vi "Main.vi"(8 "error in":errorcluster, 9 "Error Queue":refnum<queue>, 11 "Application Events":refnum<user-event>) -> (0 "error out":errorcluster)   [LabVIEW 2020, in "Display Console.lvlib"]
doc: "VI Template with default error structure"
uses:
  Display Console.lvlib
  Error/Controls/Error Message Object.ctl
  Controller/Controls/Application Modules.ctl
  Error/Controls/Error Commands.ctl
  Controller/Controls/Application Event Object.ctl
  Controller/Controls/Application Events.ctl
  Controls/Operational Loop Commands.ctl
  Controls/Event Loop Data.ctl
  Controls/Operational Loop Data.ctl
  Controller/Controller.lvlib
  Error/Error Handler.lvlib
panel:
  out "Card Read":bool
  out "Message Screen":string
  out "Current Transaction":string
  # "[Covers: UI3B]"
  # "[Covers: UI3C]"
  # "[Covers: UI3]"
  # "[Covers: UI3A]"
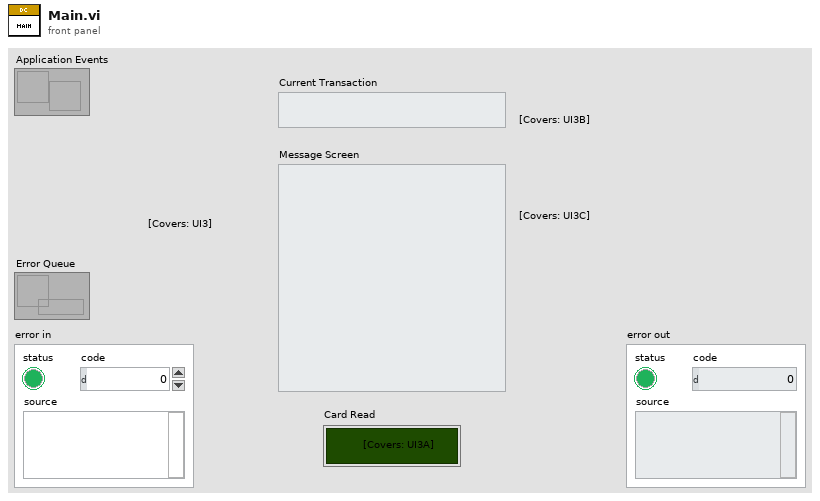
[diagram p1: front panel]
types:
  T1 = cluster{"Welcome Message":string, "Login Message":string, "Invalid Login Message":string, "Idle Message":string, "Terminate Session Message":string}
  T2 = typedef "Display Console.lvlib/Operational Loop Data.ctl" = cluster{"Current Module":T3}
  T3 = typedef "Controller.lvlib/Application Modules.ctl" = enum16{"Controller", "Error Module", "User Console", "Display Console", "Sensor Interface"}
  T4 = typedef "Display Console.lvlib/Event Loop Data.ctl" = cluster{"Current Module":T3, "Welcome Screen Messages":cluster{"Welcome Message":string, "Login Message":string, "Invalid Login Message":string, "Idle Message":string, "Terminate Session Message":string}}
  T5 = typedef "Controller.lvlib/Application Events.ctl" = enum16{"Terminate App", "Initialize", "New Transaction", "Balance Inquiry", "Balance Inquiry: Answer", "Deposit", "Deposit: Answer", "Withdrawal", "Withdrawal: Amount", "Fast Cash 50$", "Terminate Session", "Login", "Verify Account", "Invalid Login"}
  T6 = typedef "Display Console.lvlib/Operational Loop Commands.ctl" = enum16{"Shutdown"}
  T7 = enum16{"Load References", "Release References", "Get References"}
  T8 = typedef "Controller.lvlib/Controller Message Object.ctl" = cluster{"Commands":T9, "Source Module":T3, "Event Data":variant}
  T9 = typedef "Controller Commands.ctl" = enum16{"Shutdown"}
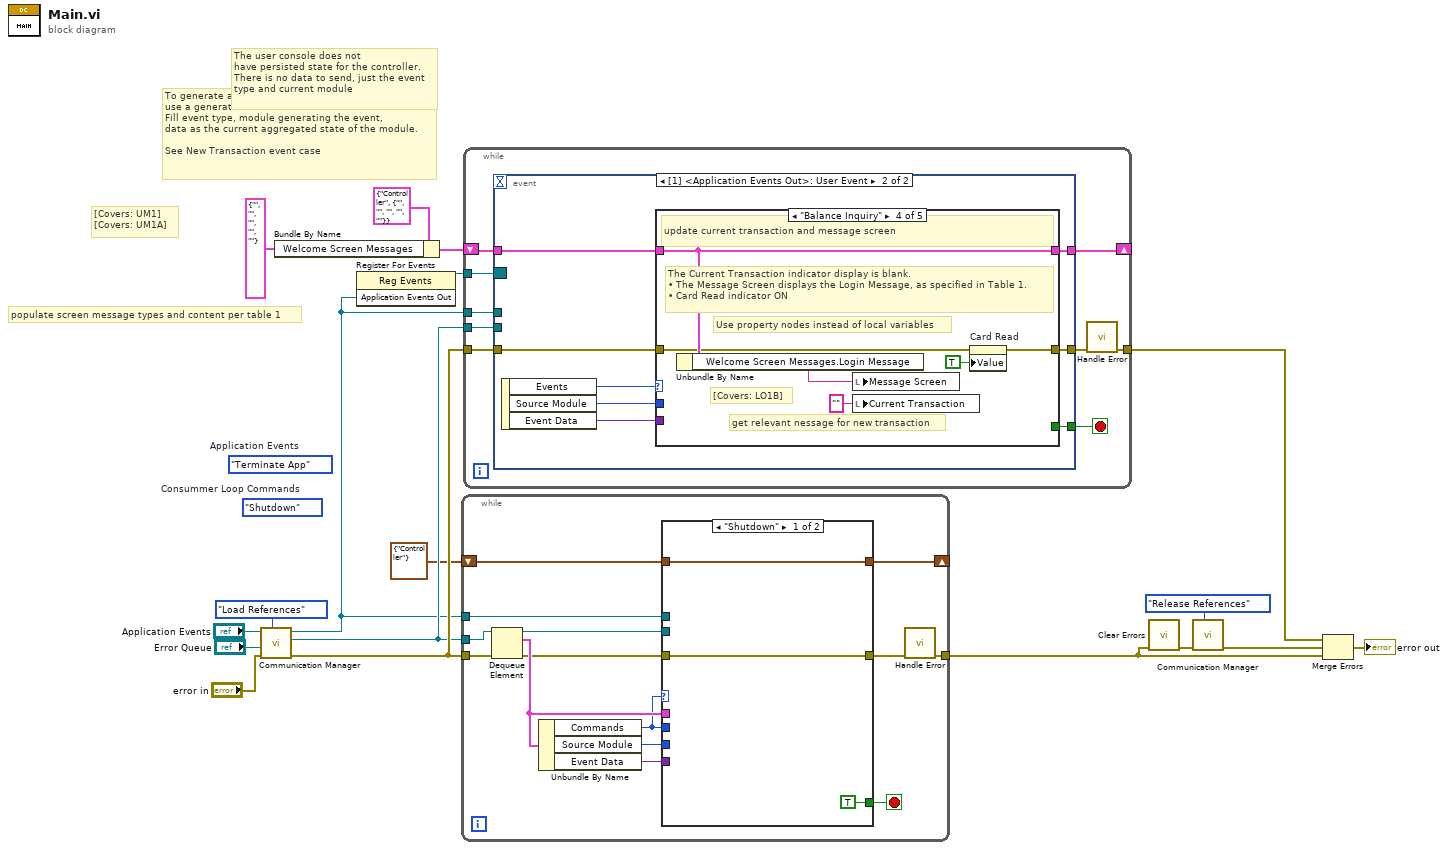
[diagram p0: block diagram]
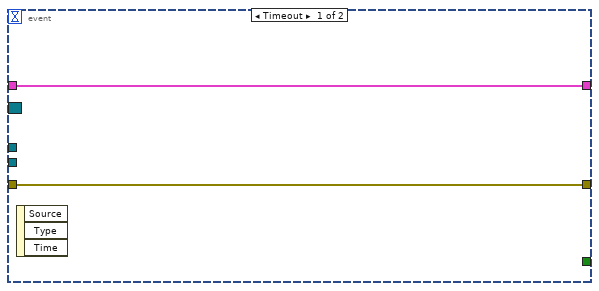
[diagram p3: hidden frame]
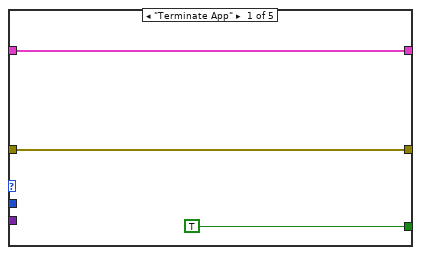
[diagram p4: hidden frame]
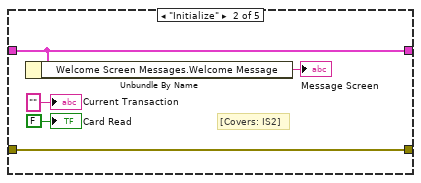
[diagram p5: hidden frame]
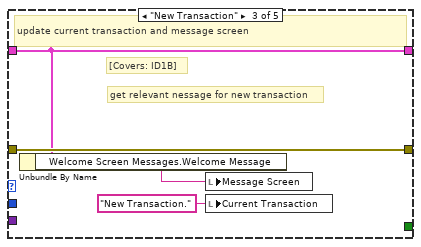
[diagram p6: hidden frame]
diagram:
  (unwired) Application_Events."Terminate App"  # Application Events
  (unwired) Operational_Loop_Commands."Shutdown"  # Consummer Loop Commands
  # "The user console does not\nhave persisted state for the controller.\nThere is no data to send, just the event\ntype and current module"
  # "To generate an event, \nuse a generate user event vi.\nFill event type, module generating the event,\ndata as the current aggregated state of the module.\n\nSee New Transaction event case"
  # "[Covers: UM1] \n[Covers: UM1A]"
  # "populate screen message types and content per table 1"
  n1 = call "Communication Manager.vi"("Mode"=T7."Load References", "error in"="error in", "Error Queue"="Error Queue", "Application Events"="Application Events") -> ("error out"=w15:errorcluster, "Module Queue Out"=w7:refnum<queue>, "Application Events Out"=w6:refnum<user-event>)  [unwired: 4 in, 1 out]
  n2 = Bundle By Name(cluster=T4 {"Current Module"=enum."Controller", "Welcome Screen Messages"={"Welcome Message"="", "Login Message"="", "Invalid Login Message"="", "Idle Message"="", "Terminate Session Message"=""}} ("Event Loop Data"), "Welcome Screen Messages"=T1 {"Welcome Message"="", "Login Message"="", "Invalid Login Message"="", "Idle Message"="", "Terminate Session Message"=""}) -> (w2:T4)
  n3 = register-events(w6) -> (reference out=w5:refnum<event-registration>)  [unwired: 2 in, 1 out]
  n4 = while {
    tunnel: w15 -> [w31]
    tunnel: w7 -> [w30]
    tunnel: [w32] -> w9
    tunnel: w6 -> [w23]
    shift-right: [w20] -> _
    shift-left: T2 {"Current Module"=enum."Controller"} ("Operational Loop Data") -> [w21]
    stop <- w24 stop-if-true
    n5 = Dequeue Element(queue=w30, error in (no error)=w31) -> (queue out=w22:refnum<queue>, element=w28:T8, error out=w19:errorcluster)  [unwired: 1 in, 1 out]
    n6 = Unbundle By Name(w28) -> ("Commands"=w25:T9, "Source Module"=w27:T3, "Event Data"=w26:variant)
    n7 = case shown="\"Shutdown\"" w25 {
      tunnel: w19 -> [w35 w37]
      tunnel: [w35 w37] -> w29
      tunnel: w28 -> [_ _]
      tunnel: w25 -> [_ _]
      tunnel: w27 -> [_ _]
      tunnel: w26 -> [_ _]
      tunnel: [TRUE _] -> w24
      tunnel: w23 -> [_ _]
      tunnel: w22 -> [_ _]
      tunnel: w21 -> [w33 w36]
      tunnel: [w33 w36] -> w20
      frame "Shutdown" {
      }
      frame Default {
      }
    }
    n8 = call "Handle Error.vi"("error in"=w29) -> ("error out"=w32:errorcluster)  [unwired: 10 in]
  }
  n9 = while {
    tunnel: w15 -> [w45]
    tunnel: w6 -> [w44]
    tunnel: [w46] -> w13
    tunnel: w7 -> [w43]
    tunnel: w5 -> [w42]
    shift-right: [w39] -> _
    shift-left: w2 -> [w38]
    stop <- w40 stop-if-true
    n10 = event shown="[1] <Application Events Out>: User Event" {
      selector: w42 -> [_ _]
      dyn-events: _ -> [_ _]
      timeout: _ -> [_ _]
      tunnel: w45 -> [w48 w55]
      tunnel: w44 -> [_ _]
      tunnel: w43 -> [_ _]
      tunnel: [w48 w56] -> w41
      tunnel: [_ w51] -> w40
      tunnel: [w47 w50] -> w39
      tunnel: w38 -> [w47 w49]
      event Timeout {
        n11 = event-data() -> ()  [unwired: 1 in, 3 out]
      }
      event User Event {
        n12 = event-data() -> ("Events"=w54:T5, "Source Module"=w53:T3, "Event Data"=w52:variant)  [unwired: 1 in]
        n13 = case shown="\"Balance Inquiry\"" w54 {
          tunnel: [w59 w64 w68 w70 w76] -> w56
          tunnel: w55 -> [w59 w64 w68 w71 w76]
          tunnel: w53 -> [_ _ _ _ _]
          tunnel: w52 -> [_ _ _ _ _]
          tunnel: [TRUE _ _ _ _] -> w51
          tunnel: [w57 w61 w67 w74 w75] -> w50
          tunnel: w49 -> [w57 w61 w67 w74 w75]
          frame "Terminate App" {
          }
          frame "Initialize" {
            # "[Covers: IS2]"
            n14 = Unbundle By Name(w61) -> ("Welcome Screen Messages.Welcome Message"=→"Message Screen":string)
            "Current Transaction" <- "" ("Current Transaction")
            "Card Read" <- FALSE ("Card Read")
          }
          frame "New Transaction" {
            # "[Covers: ID1B]"
            # "get relevant nessage for new transaction"
            # "update current transaction and message screen"
            n15 = Unbundle By Name(w67) -> ("Welcome Screen Messages.Welcome Message"=w65:string)
            n16 = local write "Message Screen"(w65) -> ()
            n17 = local write "Current Transaction"("New Transaction." ("Current Transaction")) -> ()
          }
          frame "Balance Inquiry" {
            # "[Covers: LO1B]"
            # "Use property nodes instead of local variables"
            # "The Current Transaction indicator display is blank.\n• The Message Screen displays the Login Message, as specified in Table 1.\n• Card Read indicator ON"
            # "get relevant nessage for new transaction"
            # "update current transaction and message screen"
            n18 = Unbundle By Name(w74) -> ("Welcome Screen Messages.Login Message"=w72:string)
            n19 = local write "Message Screen"(w72) -> ()
            n20 = local write "Current Transaction"("" ("Current Transaction")) -> ()
            n21 = property on="Card Read" class="Bool (strict)"(error in=w71, "Value"=TRUE ("Card Read")) -> (error out=w70:errorcluster)  [unwired: 1 in, 1 out]
          }
          frame Default {
          }
        }
      }
    }
    n22 = call "Handle Error.vi"("error in"=w41) -> ("error out"=w46:errorcluster)  [unwired: 10 in]
  }
  n23 = call <vilib>:"Clear Errors.vi"("error in (no error)"=w9) -> ("error out"=w12:errorcluster)  [unwired: 5 in, 1 out]
  n24 = call "Communication Manager.vi"("Mode"=T7."Release References", "error in"=w12) -> ("error out"=w8:errorcluster)  [unwired: 6 in, 3 out]
  n25 = Merge Errors(w13, w8, w9) -> (→"error out":errorcluster)
